vi "host.vi"() -> ()   [LabVIEW 2010]
uses:
  fpga_vi_ref.ctl
  <vilib>/userDefined/High Color/nirio_resource_hc.ctl
  <vilib>/rvi/interface/nirviOpenFPGA/nirviOpenFPGA.xnode
  FPGA Bitfiles/FPGATest_FPGATarget_test_60EC0474.lvbitx
  <vilib>/rvi/ClientSDK/nirviWhatTheDeviceIsDoing.ctl
  <vilib>/rvi/interface/nirviReadWriteControl/nirviReadWriteControl.xnode
  <vilib>/rvi/interface/common/niFpgaNodeNameForErrorReporting.ctl
  <vilib>/rvi/errors/niLvFpgaWhatHappensToTopLevelVI.ctl
  <vilib>/rvi/interface/nirviCloseFPGA/nirviCloseFPGA.xnode
  <vilib>/FPGAPlugInAG/PXI-7813R/niLvFpga_Open_PXI-7813R.vi
  <vilib>/Utility/error.llb/Error Cluster From Error Code.vi
  <vilib>/rvi/errors/niLvFpgaAdjustHostInterfaceError.vi
  <vilib>/FPGAPlugInAG/PXI-7813R/niLvFpga_Close_PXI-7813R.vi
  NiFpgaLv.dll
panel:
  out "FPGA VI Reference Out":T1
  out "out":i16
  in  "In":i16
  in  "stop":bool
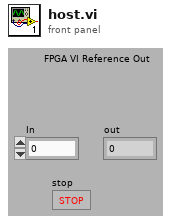
[diagram p1: front panel]
types:
  T1 = typedef "fpga_vi_ref.ctl" = refnum<k20>
  T2 = typedef "nirio_resource_hc.ctl" = tag
  T3 = typedef "niFpgaNodeNameForErrorReporting.ctl" = enum16{"Open FPGA VI Reference", "Read/Write Control", "Invoke Method: Abort", "Invoke Method: Acknowledge IRQ", "Invoke Method: Download", "Invoke Method: FIFO.Configure", "Invoke Method: FIFO.Read", "Invoke Method: FIFO.Start", "Invoke Method: FIFO.Stop", "Invoke Method: FIFO.Write", "Invoke Method: Reset", "Invoke Method: Run", "Invoke Method: Wait on IRQ", "Close FPGA VI Reference"}
  T4 = typedef "niLvFpgaWhatHappensToTopLevelVI.ctl" = enum16{"top level VI scripted behind XNode", "top level VI inlined behind XNode"}
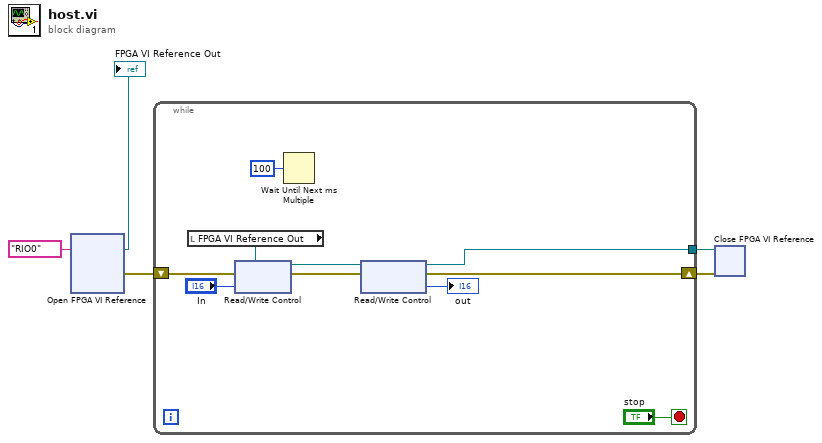
[diagram p0: block diagram]
diagram:
  n1 = xnode "Open FPGA VI Reference"("resource name"=T2 "RIO0") -> ("FPGA VI Reference Out"=→"FPGA VI Reference Out":T1, "error out"=w5:errorcluster)  [unwired: 1 in]
  n2 = while {
    shift-right: [w9] -> w4
    shift-left: w5 -> [w15]
    tunnel: [w11] -> w3
    stop <- "stop" stop-if-true
    n3 = local read "FPGA VI Reference Out"() -> (w6:T1)
    n4 = xnode "Read/Write Control"("FPGA VI Reference In"=w6, "error in"=w15, "Numeric"="In") -> ("FPGA VI Reference Out"=w12:T1, "error out"=w10:errorcluster)
    n5 = Wait Until Next ms Multiple(millisecond multiple=u32 100) -> ()  [unwired: 1 out]
    n6 = xnode "Read/Write Control"("FPGA VI Reference In"=w12, "error in"=w10) -> ("FPGA VI Reference Out"=w11:T1, "error out"=w9:errorcluster, "Numeric 2"=→"out":i16)
  }
  n7 = xnode "Close FPGA VI Reference"("FPGA VI Reference In"=w3, "error in"=w4) -> ()  [unwired: 1 out]
